vi "Query_SubVIs-某型振动实验台测试系统.vi"(8 "Error":errorcluster) -> (0 "Error":errorcluster)   [LabVIEW 2011]
doc: "Use this template to build a VI to use as a subVI."
uses:
  Ctrls/ana data.ctl
panel:
  out "units":string[](array[string])
  out "粉尘特性":T1
  out "测试条件out":T2
  in  "Tempre Chart 2":waveform(dbl)
  in  "Tempre Chart":waveform(dbl)
  in  "Exit":bool caption="返回"
  in  "Report":bool caption="生成报表"
  in  "Open":bool caption="读取"
  in  "Temp":T3={"Vibr Chn Name"=[], "Analysis Chn Number"=0, "Index Vibration Waveform"={"t0"=timestamp(0 s since 1904-01-01), "dt"=1.0, "Y"=[]}, "Report Infomation"={"Test Name"="", "Tester"="", "Tempre Chart"=refnum, "Apli-Fre"=refnum, "Phase-Fre"=refnum, "Raw Data"=refnum}, "Vibr Apli - Fre"=[], "Vibr Phase - Fre"=[], "Error"={"status"=FALSE, "code"=0, "source"=""}, "Read Chan Name"="", "Test Info"={"Test Name"="", "Tester"=""}, "test data"=[{"t0"=timestamp(0 s since 1904-01-01), "dt"=1.0, "Y"=[]}, {"t0"=timestamp(0 s since 1904-01-01), "dt"=1.0, "Y"=[]}, {"t0"=timestamp(0 s since 1904-01-01), "dt"=1.0, "Y"=[]}, {"t0"=timestamp(0 s since 1904-01-01), "dt"=0.001, "Y"=[]}], "测试头文件"={"ch"=[{"pmax"="", "dp/dt"=""}, {"pmax"="", "dp/dt"=""}, {"pmax"="", "dp/dt"=""}, {"pmax"="", "dp/dt"=""}, {"pmax"="无", "dp/dt"="无"}], "测试环境"=""}, "CAl VAlUE"={"max_t"=[], "max_V"=[], "start_t"=[], "start_V"=[], "distance"=[], "unit"="m"}}
  out "Tester":string caption="实验人"
  out "Test Name":string caption="实验名称"
  in  "Tab Control":enum32{"信号原始数据", "幅频波形", "相频波形"}(tab)
  out "start point":string
  out "high point":string
  in  "unit":enum16{"m", "Km"}(ring) caption="单位："
  in  "print":bool
  out "max_t1":dbl caption="1点至2点"
  out "start_t1":dbl caption="1点至2点"
  out "max_V2":dbl caption="1点至3点"
  out "max_V1":dbl caption="1点至2点"
  in  "T_AN":bool
  out "Raw Data Chart":waveform(dbl)[](graph)
  in  "Tree":string(tree)="PXI-4472/ai0"
  in  "平均时间(S)":dbl=0.002
  in  "Radio Buttons":enum32{"原始数据", "处理数据"}(radio)
  in  "1点至2点距离":dbl=11.0
  in  "1点至3点距离":dbl=12.0
  out "max_t2":dbl caption="1点至3点"
  out "start_t2":dbl caption="1点至3点"
  out "start_V1":dbl caption="1点至2点"
  out "start_V2":dbl caption="1点至3点"
  out "high point 2":string
  out "start point 2":string
  out "Apli-Fre":cluster{dbl, dbl}[](graph)
  out "Phase-Frequency":cluster{dbl, dbl}[](graph)
  # "数据查询与分析"
  # "最高点\n  延迟时间："
  # "s"
  # "s"
  # "最高点\n   传播速度："
  # "开始点\n    延迟时间："
  # "s"
  # "s"
  # "开始点\n   传播速度："
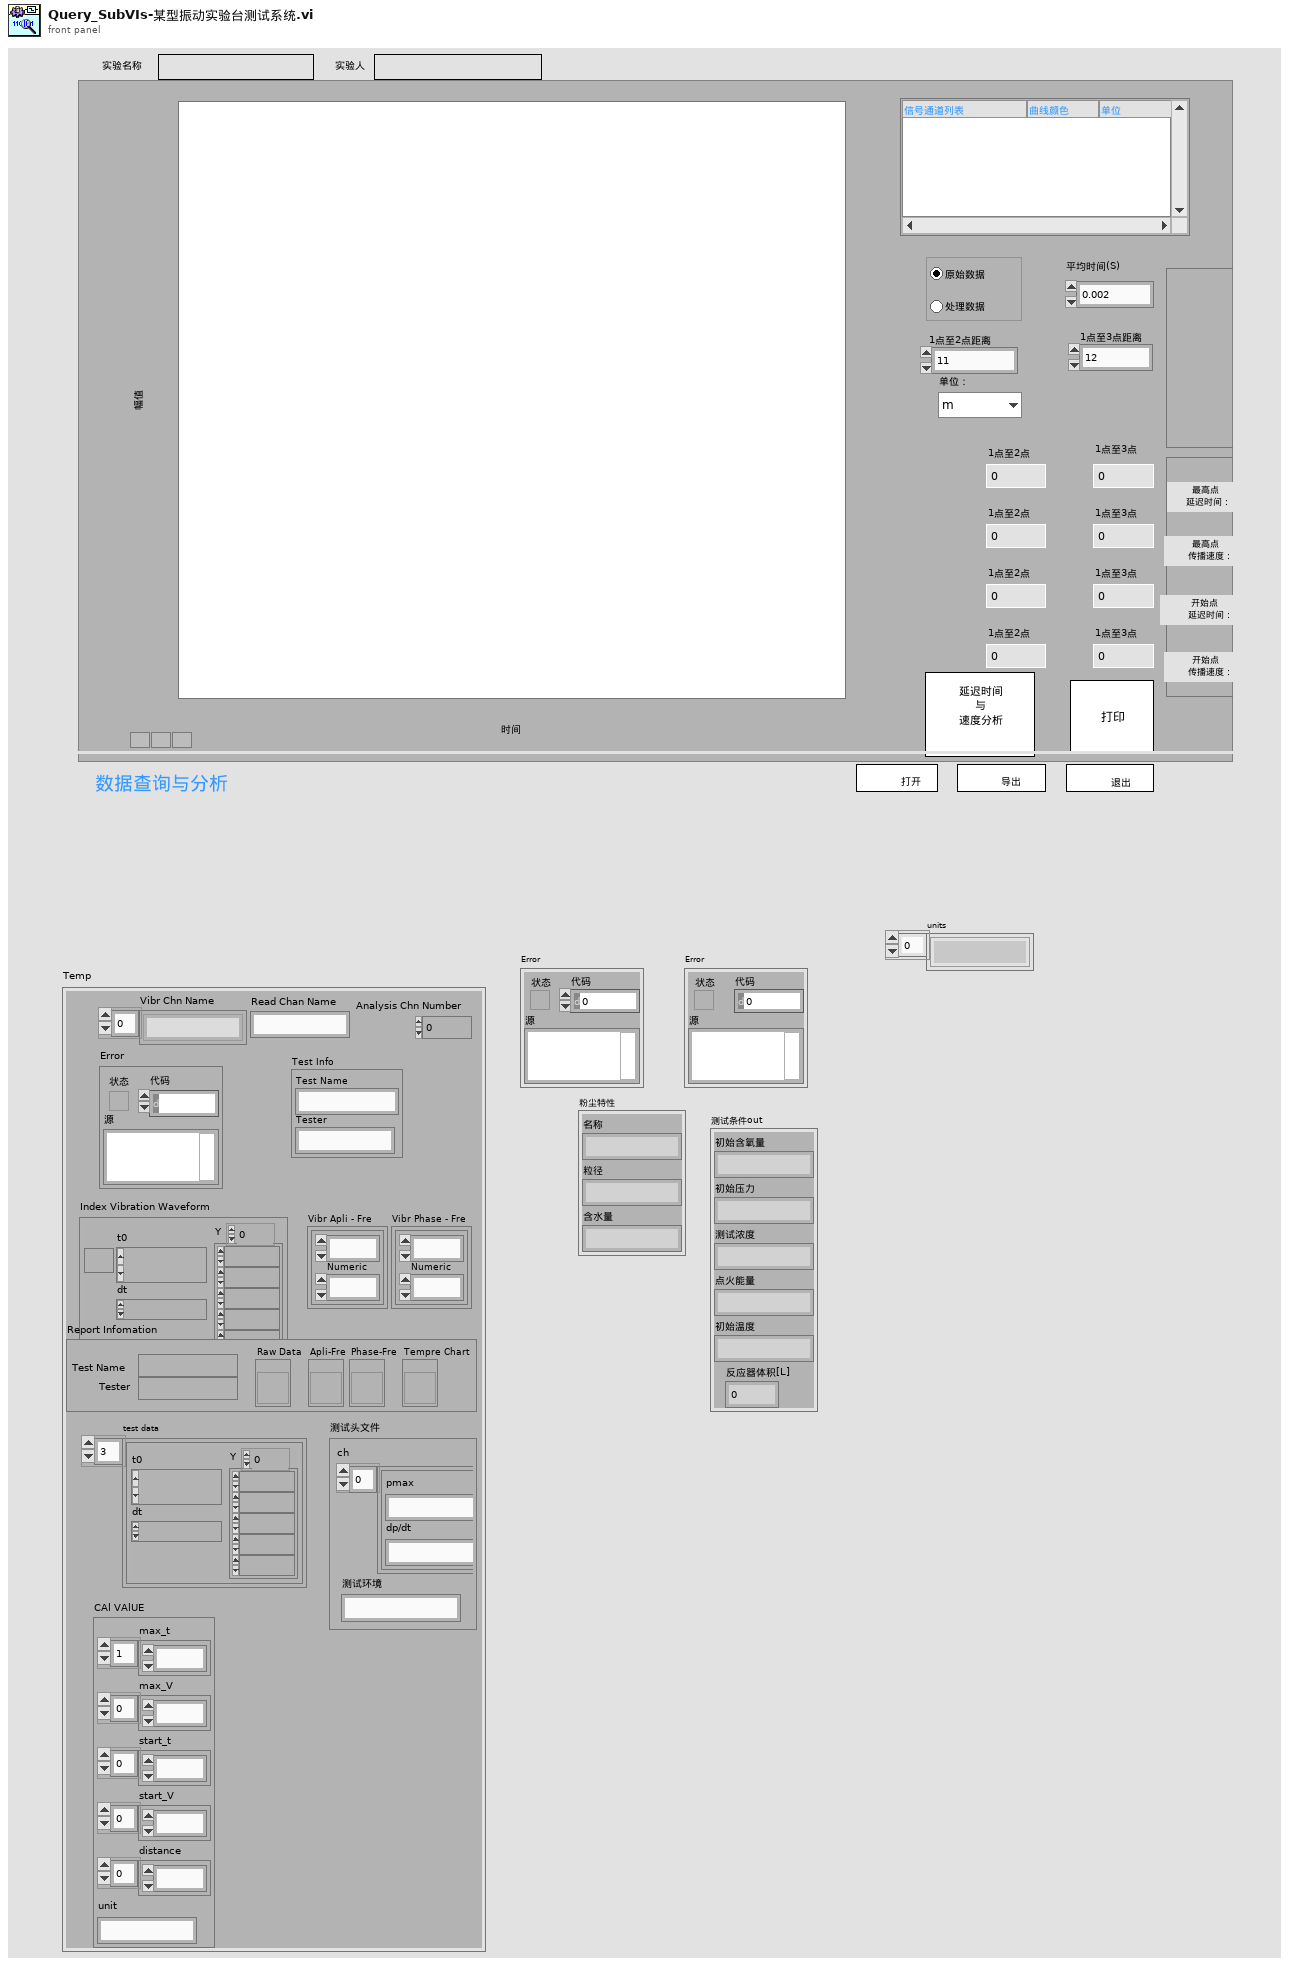
[diagram p1: front panel]
types:
  T1 = typedef "粉尘特性.ctl" = cluster{"名称":string, "粒径":string, "含水量":string}
  T2 = typedef "测试条件.ctl" = cluster{"初始含氧量":string, "初始压力":string, "测试浓度":string, "点火能量":string, "初始温度":string, "反应器体积[L]":dbl}
  T3 = typedef "ana data.ctl" = cluster{"Vibr Chn Name":string[], "Analysis Chn Number":i32, "Index Vibration Waveform":waveform(dbl), "Report Infomation":cluster{"Test Name":string, "Tester":string, "Tempre Chart":refnum<vi>, "Apli-Fre":refnum<vi>, "Phase-Fre":refnum<vi>, "Raw Data":refnum<vi>}, "Vibr Apli - Fre":cluster{dbl, "Numeric":dbl}[], "Vibr Phase - Fre":cluster{dbl, "Numeric":dbl}[], "Error":errorcluster, "Read Chan Name":string, "Test Info":cluster{"Test Name":string, "Tester":string}, "test data":waveform(dbl)[], "测试头文件":cluster{"ch":cluster{"pmax":string, "dp/dt":string}[], "测试环境":string}, "CAl VAlUE":cluster{"max_t":dbl[], "max_V":dbl[], "start_t":dbl[], "start_V":dbl[], "distance":dbl[], "unit":string}}
  T4 = typedef "Enum Query_Ctrls-某型振动实验台测试系统.ctl" = enum16{"Initialize", "No Action", "Open TDMS File", "Read Raw Data", "Analyze Data", "Display Data", "Generate Report", "computer timer", "Error Handle", "Exit"}
  T5 = typedef "Enum File IO - FGV(V)_Ctrls-某型振动实验台测试系统.ctl" = enum16{"New", "Open", "Write Info", "Write Data", "Read Info", "Read Chan Names", "Read Data", "Close", "None"}
  T6 = typedef "imagedata.ctl" = cluster{"image type":i32, "image depth":i32, "image":u8[], "mask":u8[], "colors":u32[], "Rectangle":cluster{"left":i16, "top":i16, "right":i16, "bottom":i16}}
  T7 = cluster{"max_t":dbl[], "max_V":dbl[], "start_t":dbl[], "start_V":dbl[]}
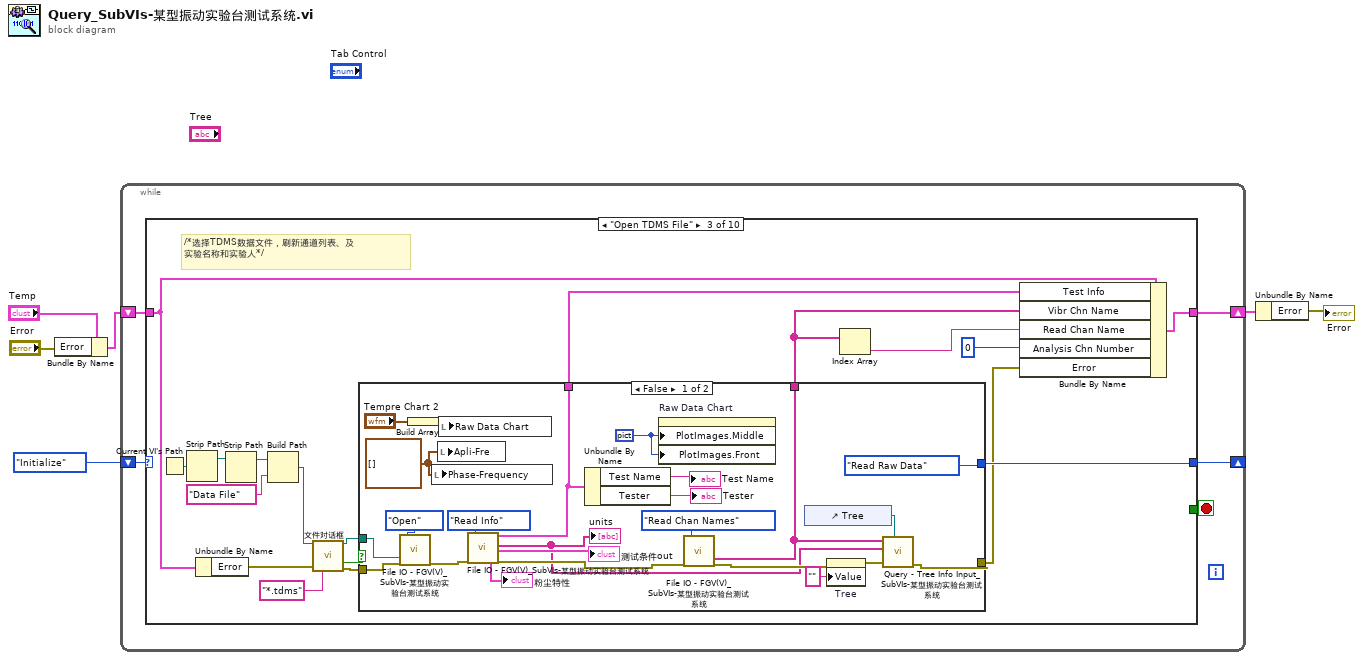
[diagram p0: block diagram]
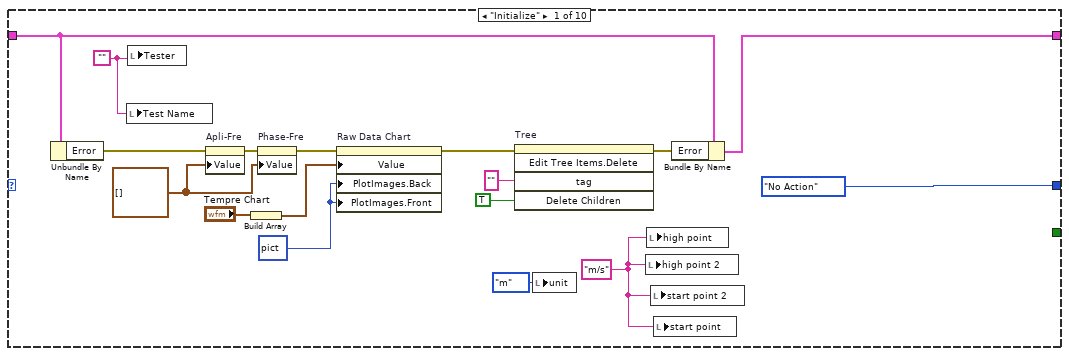
[diagram p2: hidden frame]
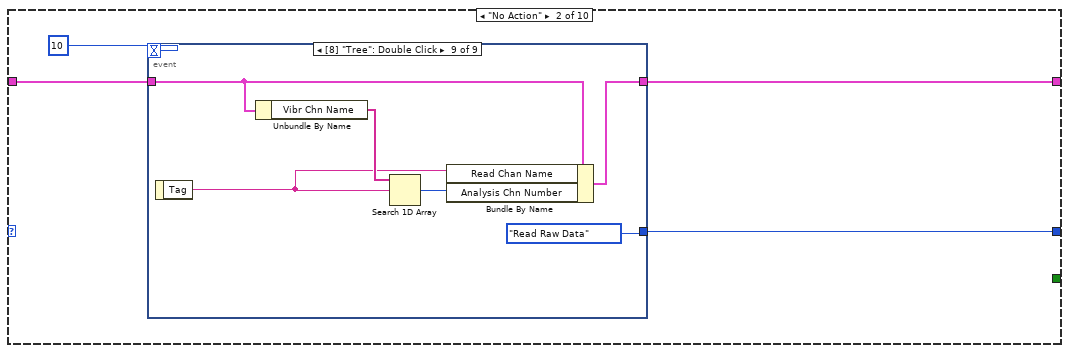
[diagram p3: hidden frame]
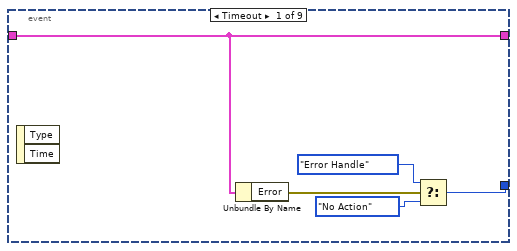
[diagram p4: hidden frame]
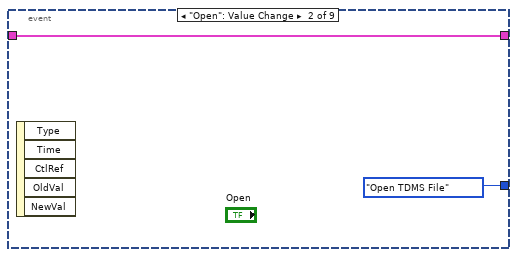
[diagram p5: hidden frame]
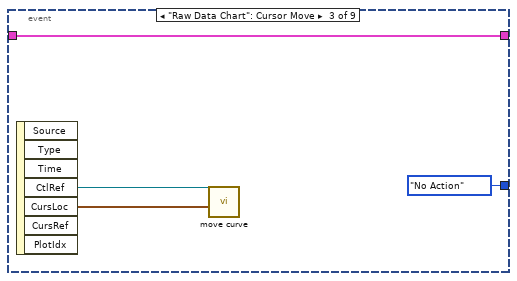
[diagram p6: hidden frame]
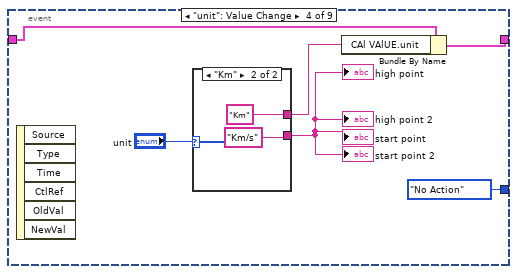
[diagram p7: hidden frame]
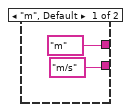
[diagram p8: hidden frame]
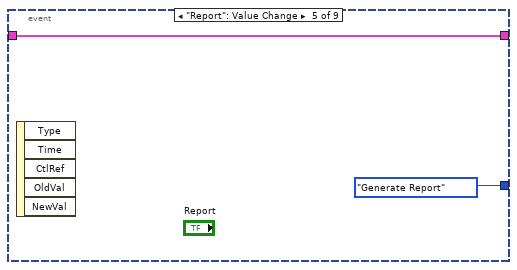
[diagram p9: hidden frame]
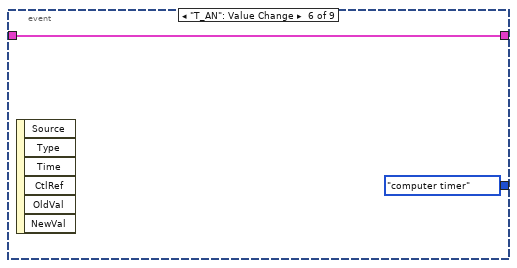
[diagram p10: hidden frame]
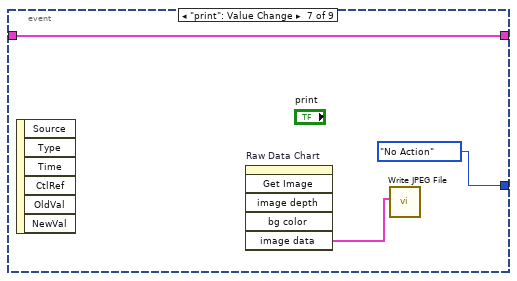
[diagram p11: hidden frame]
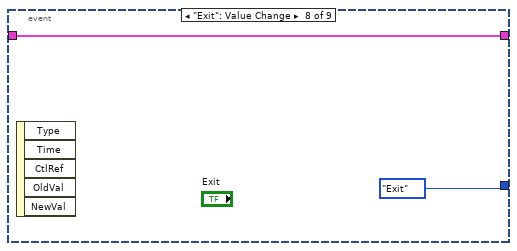
[diagram p12: hidden frame]
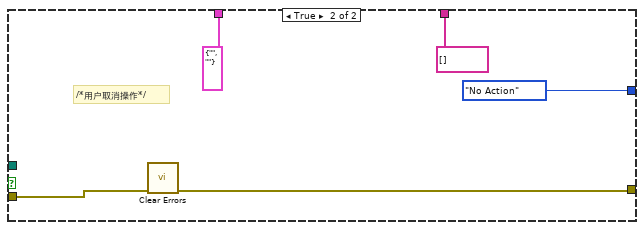
[diagram p13: hidden frame]
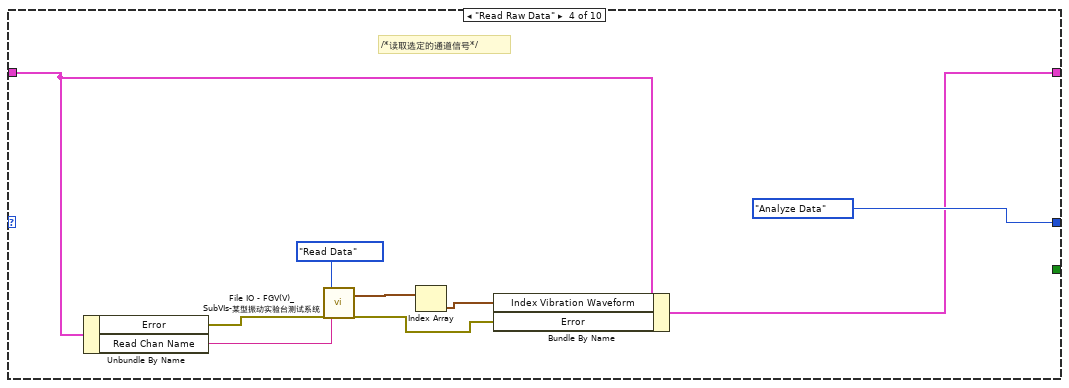
[diagram p14: hidden frame]
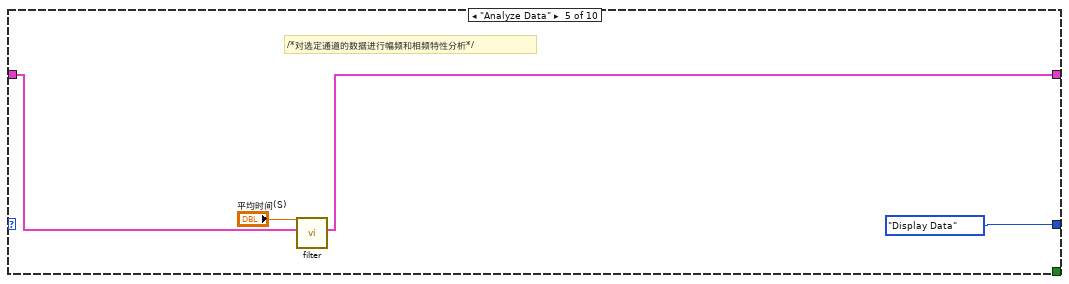
[diagram p15: hidden frame]
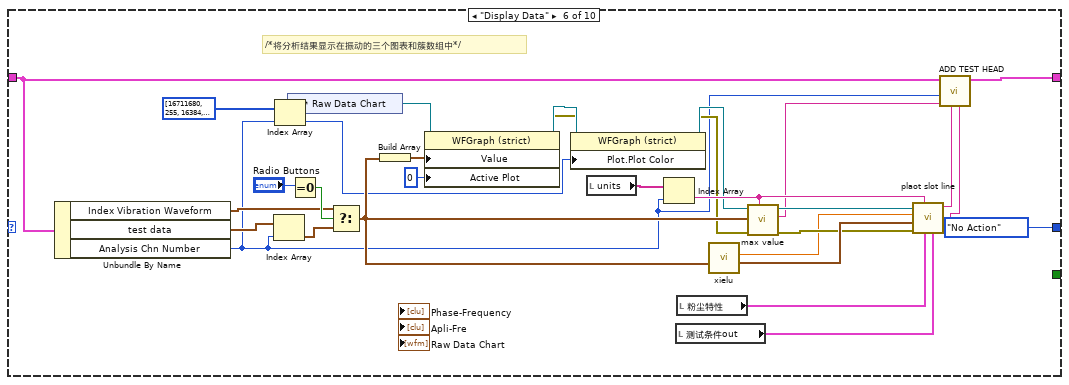
[diagram p16: hidden frame]
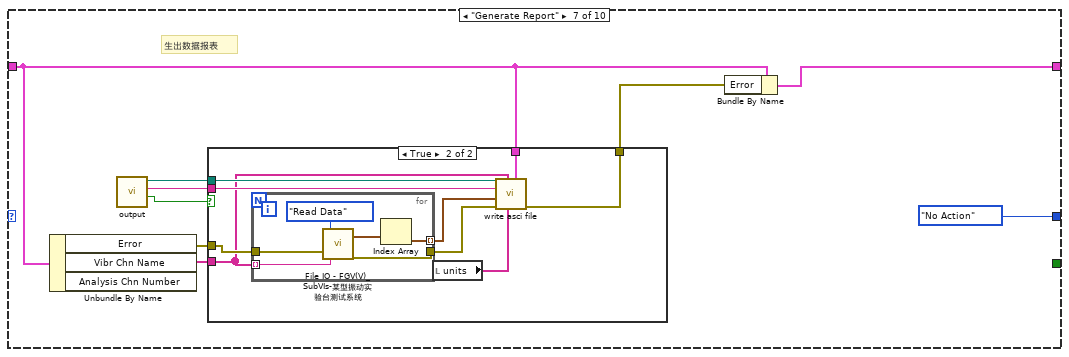
[diagram p17: hidden frame]
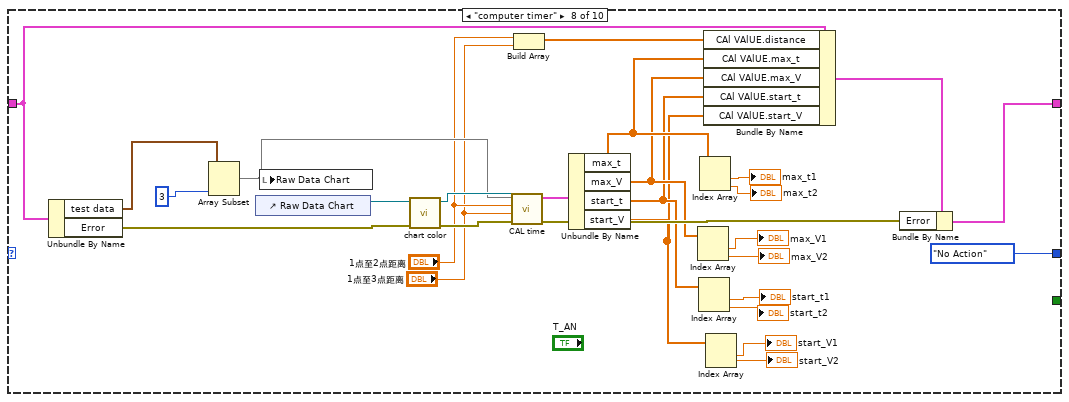
[diagram p19: hidden frame]
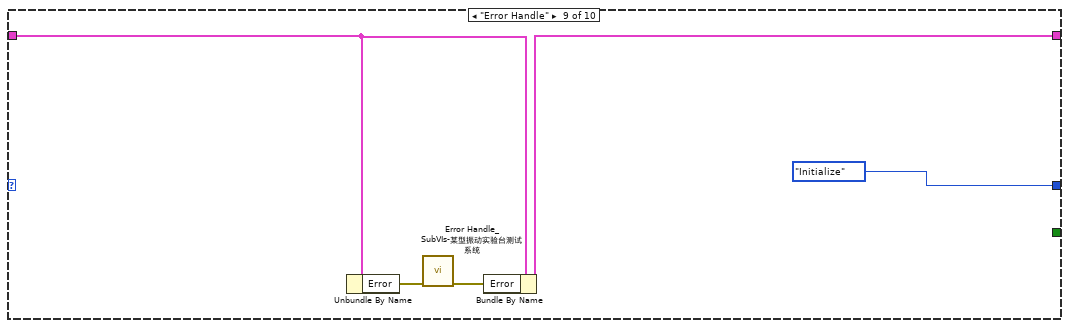
[diagram p20: hidden frame]
diagram:
  n1 = Bundle By Name(cluster="Temp", "Error"="Error") -> (w3:T3)
  n2 = while {
    shift-right: [w10] -> _
    shift-left: Enum_Query_Ctrls-某型振动实验台测试系统."Initialize" ("Enum") -> [w11]
    shift-right: [w7] -> w2
    shift-left: w3 -> [w8]
    stop <- w9 stop-if-true
    n3 = case shown="\"Open TDMS File\"" w11 {
      tunnel: [Enum_Query_Ctrls-某型振动实验台测试系统."No Action" ("Enum") w31 w77 Enum_Query_Ctrls-某型振动实验台测试系统."Analyze Data" ("Enum") Enum_Query_Ctrls-某型振动实验台测试系统."Display Data" ("Enum") Enum_Query_Ctrls-某型振动实验台测试系统."No Action" ("Enum") Enum_Query_Ctrls-某型振动实验台测试系统."No Action" ("Enum") Enum_Query_Ctrls-某型振动实验台测试系统."No Action" ("Enum") Enum_Query_Ctrls-某型振动实验台测试系统."Initialize" ("Enum") Enum_Query_Ctrls-某型振动实验台测试系统."Exit" ("Enum")] -> w10
      tunnel: [_ _ _ _ _ _ _ _ _ TRUE] -> w9
      tunnel: w8 -> [w22 w30 w72 w121 w127 w134 w159 w191 w212 w216]
      tunnel: [w20 w29 w76 w123 w126 w133 w166 w209 w211 w216] -> w7
      frame "Initialize" {
        w14 = picture data[5B] ("曲线图像:前景")
        w12 = "m/s" ("Tag")
        w24 = cluster{dbl, dbl}[] [] ("Aplitude-Frequency")
        w25 = ""
        n4 = Unbundle By Name(w22) -> ("Error"=w23:errorcluster)
        n5 = local write "Test Name"(w25) -> ()
        n6 = local write "Tester"(w25) -> ()
        n7 = property on="Apli-Fre" class="XYGraph (strict)"(error in=w23, "Value"=w24) -> (error out=w27:errorcluster)  [unwired: 1 in, 1 out]
        n8 = Build Array("Tempre Chart") -> (w15:waveform(dbl)[])
        n9 = property on="Phase-Fre" class="XYGraph (strict)"(error in=w27, "Value"=w24) -> (error out=w26:errorcluster)  [unwired: 1 in, 1 out]
        n10 = property on="Raw Data Chart" class="WFGraph (strict)"(error in=w26, "Value"=w15, "PlotImages.Back"=w14, "PlotImages.Front"=w14) -> (error out=w19:errorcluster)  [unwired: 1 in, 1 out]
        n11 = invoke on="Tree" class="Tree (严格)" method="Edit Tree Items.Delete"(error in=w19, "tag"="" ("Tag"), "Delete Children"=TRUE ("Delete Children?")) -> (error out=w21:errorcluster)  [unwired: 2 in, 4 out]
        n12 = local write "unit"(enum16{"m", "Km"}."m" ("unit")) -> ()
        n13 = local write "high point 2"(w12) -> ()
        n14 = local write "high point"(w12) -> ()
        n15 = local write "start point 2"(w12) -> ()
        n16 = local write "start point"(w12) -> ()
        n17 = Bundle By Name(cluster=w22, "Error"=w21) -> (w20:T3)
      }
      frame "No Action" {
        n18 = event shown="[8] \"Tree\": Double Click" {
          selector: _ -> [_ _ _ _ _ _ _ _ _]
          dyn-events: _ -> [_ _ _ _ _ _ _ _ _]
          timeout: 10 -> [_ _ _ _ _ _ _ _ _]
          tunnel: [w35 Enum_Query_Ctrls-某型振动实验台测试系统."Open TDMS File" ("Enum") Enum_Query_Ctrls-某型振动实验台测试系统."No Action" ("Enum") Enum_Query_Ctrls-某型振动实验台测试系统."No Action" ("Enum") Enum_Query_Ctrls-某型振动实验台测试系统."Generate Report" ("Enum") Enum_Query_Ctrls-某型振动实验台测试系统."computer timer" ("Enum") Enum_Query_Ctrls-某型振动实验台测试系统."No Action" ("Enum") Enum_Query_Ctrls-某型振动实验台测试系统."Exit" ("Enum") Enum_Query_Ctrls-某型振动实验台测试系统."Read Raw Data" ("Enum")] -> w31
          tunnel: w30 -> [w34 w38 w43 w46 w54 w57 w60 w61 w65]
          tunnel: [w34 w38 w43 w45 w54 w57 w60 w61 w64] -> w29
          event Timeout {
            n19 = event-data() -> ()  [unwired: 3 out]
            n20 = Unbundle By Name(w34) -> ("Error"=w33:errorcluster)
            n21 = Select(t=Enum_Query_Ctrls-某型振动实验台测试系统."Error Handle" ("Enum"), s=w33, f=Enum_Query_Ctrls-某型振动实验台测试系统."No Action" ("Enum")) -> (s? t:f=w35:T4)
          }
          event "Open": Value Change {
            n22 = event-data() -> ()  [unwired: 6 out]
          }
          event "Raw Data Chart": Cursor Move {
            n23 = event-data() -> ("CtlRef"=w41:refnum<vi>, "CursLoc"=w40:cluster{"X":dbl, "Y":dbl})  [unwired: 6 out]
            n24 = call "move curve.vi"("XY"=w40, "引用"=w41) -> ()  [unwired: 1 in, 9 out]
          }
          event "unit": Value Change {
            n25 = event-data() -> ()  [unwired: 7 out]
            n26 = case shown="\"Km\"" "unit" {
              tunnel: ["m/s" "Km/s"] -> w47
              tunnel: ["m" "Km"] -> w44
              frame "m", Default {
              }
              frame "Km" {
              }
            }
            "high point" <- w47
            "start point" <- w47
            "high point 2" <- w47
            "start point 2" <- w47
            n27 = Bundle By Name(cluster=w46, "CAl VAlUE.unit"=w44) -> (w45:T3)
          }
          event "Report": Value Change {
            n28 = event-data() -> ()  [unwired: 6 out]
          }
          event "T_AN": Value Change {
            n29 = event-data() -> ()  [unwired: 7 out]
          }
          event "print": Value Change {
            n30 = event-data() -> ()  [unwired: 7 out]
            n31 = invoke on="Raw Data Chart" class="WFGraph (严格)" method="Get Image"() -> ("image data"=w59:T6)  [unwired: 6 in, 5 out]
            n32 = call <vilib>:"Write JPEG File.vi"("image data"=w59) -> ()  [unwired: 2 in, 9 out]
          }
          event "Exit": Value Change {
            n33 = event-data() -> ()  [unwired: 6 out]
          }
          event "Tree": Double Click {
            n34 = event-data() -> ("Tag"=w63:string)  [unwired: 1 out]
            n35 = Unbundle By Name(w65) -> ("Vibr Chn Name"=w67:string[])
            n36 = Search 1D Array(1D array=w67, element=w63) -> (index of element=w66:i32)  [unwired: 1 out]
            n37 = Bundle By Name(cluster=w65, "Read Chan Name"=w63, "Analysis Chn Number"=w66) -> (w64:T3)
          }
        }
      }
      frame "Open TDMS File" {
        # "/*选择TDMS数据文件，刷新通道列表、及\n实验名称和实验人*/"
        n38 = Current VI's Path() -> (path=w82:path)
        n39 = Strip Path(path=w82) -> (stripped path=w83:path)  [unwired: 1 out]
        n40 = Unbundle By Name(w72) -> ("Error"=w74:errorcluster)
        n41 = Strip Path(path=w83) -> (stripped path=w81:path)  [unwired: 1 out]
        n42 = Build Path(base path=w81, name or relative path="Data File") -> (appended path=w78:path)
        n43 = call "文件对话框"("start path"=w78, "error in"=w74, "pattern (all files)"="*.tdms") -> ("selected path"=w86:path, "cancelled"=w84:bool, "error out"=w85:errorcluster)  [unwired: 4 in, 6 out]
        n44 = case shown="False" w84 {
          tunnel: w86 -> [w101 _]
          tunnel: [w87 w115] -> w73
          tunnel: w85 -> [w100 w114]
          tunnel: [w105 string[] [] ("Vibration Channel Name Output")] -> w70
          tunnel: [Enum_Query_Ctrls-某型振动实验台测试系统."Read Raw Data" ("Enum") Enum_Query_Ctrls-某型振动实验台测试系统."No Action" ("Enum")] -> w77
          tunnel: [w96 cluster{"Test Name":string, "Tester":string} {"Test Name"="", "Tester"=""} ("Name")] -> w75
          frame False {
            w91 = picture data[5B] ("曲线图像:背景")
            w102 = cluster{dbl, dbl}[] [] ("Aplitude-Frequency")
            n45 = call "File IO - FGV(V)_SubVIs-某型振动实验台测试系统.vi"("文件路径"=w101, "error in"=w100, "Operation"=Enum_File_IO_-_FGV(V)_Ctrls-某型振动实验台测试系统."Open") -> ("error out"=w98:errorcluster)  [unwired: 7 in, 9 out]
            n46 = Build Array("Tempre Chart 2") -> (w94:waveform(dbl)[])
            n47 = local write "Phase-Frequency"(w102) -> ()
            n48 = local write "Apli-Fre"(w102) -> ()
            n49 = local write "Raw Data Chart"(w94) -> ()
            n50 = call "File IO - FGV(V)_SubVIs-某型振动实验台测试系统.vi"("error in"=w98, "Operation"=Enum_File_IO_-_FGV(V)_Ctrls-某型振动实验台测试系统."Read Info") -> ("粉尘特性 out"=→"粉尘特性":T1, "Test Info"=w96:cluster{"Test Name":string, "Tester":string}, "units"=w89:string[], "测试条件out"=→"测试条件out":T2, "error out"=w99:errorcluster)  [unwired: 8 in, 5 out]
            "units" <- w89
            n51 = Unbundle By Name(w96) -> ("Test Name"=→"Test Name":string, "Tester"=→"Tester":string)
            n52 = property on="Raw Data Chart" class="WFGraph (strict)"("PlotImages.Middle"=w91, "PlotImages.Front"=w91) -> ()  [unwired: 2 in, 2 out]
            n53 = call "File IO - FGV(V)_SubVIs-某型振动实验台测试系统.vi"("error in"=w99, "Operation"=Enum_File_IO_-_FGV(V)_Ctrls-某型振动实验台测试系统."Read Chan Names") -> ("Vibration Chan Names Out"=w105:string[], "error out"=w106:errorcluster)  [unwired: 8 in, 8 out]
            n54 = control-ref of="Tree"() -> (w88:refnum<vi>)
            n55 = property on="Tree" class="Tree (strict)"(error in=w106, "Value"="" ("Tree")) -> (error out=w90:errorcluster)  [unwired: 1 in, 1 out]
            n56 = call "Query - Tree Info Input_SubVIs-某型振动实验台测试系统.vi"("Tree引用句柄"=w88, "错误输入（无错误）"=w90, "units"=w89, "Vibration Channel Name Output"=w105) -> ("错误输出"=w87:errorcluster)  [unwired: 7 out]
          }
          frame True {
            # "/*用户取消操作*/"
            n57 = call <vilib>:"Clear Errors.vi"("error in (no error)"=w114) -> ("error out"=w115:errorcluster)  [unwired: 6 out]
          }
        }
        n58 = Index Array(array=w70) -> (element=w71:string)  [unwired: 1 in]
        n59 = Bundle By Name(cluster=w72, "Test Info"=w75, "Vibr Chn Name"=w70, "Read Chan Name"=w71, "Analysis Chn Number"=0, "Error"=w73) -> (w76:T3)
      }
      frame "Read Raw Data" {
        # "/*读取选定的通道信号*/"
        n60 = Unbundle By Name(w121) -> ("Error"=w120:errorcluster, "Read Chan Name"=w116:string)
        n61 = call "File IO - FGV(V)_SubVIs-某型振动实验台测试系统.vi"("error in"=w120, "Operation"=Enum_File_IO_-_FGV(V)_Ctrls-某型振动实验台测试系统."Read Data", "Chan"=w116) -> ("Vibration Waveform"=w118:waveform(dbl)[], "error out"=w119:errorcluster)  [unwired: 7 in, 8 out]
        n62 = Index Array(array=w118) -> (element=w122:waveform(dbl))  [unwired: 1 in]
        n63 = Bundle By Name(cluster=w121, "Index Vibration Waveform"=w122, "Error"=w119) -> (w123:T3)
      }
      frame "Analyze Data" {
        # "/*对选定通道的数据进行幅频和相频特性分析*/"
        n64 = call "filter.vi"("Temp"=w127, "averaging time"="平均时间(S)") -> ("Temp out"=w126:T3)  [unwired: 2 in, 7 out]
      }
      frame "Display Data" {
        # "/*将分析结果显示在振动的三个图表和簇数组中*/"
        n65 = Unbundle By Name(w134) -> ("Index Vibration Waveform"=w156:waveform(dbl), "test data"=w155:waveform(dbl)[], "Analysis Chn Number"=w132:i32)
        n66 = Index Array(array=w155, index=w132) -> (element=w154:waveform(dbl))
        n67 = Index Array(array=u32[] [16711680, 255, 16384, 4194432, 16750848], index=w132) -> (element=w139:u32)
        n68 = control-ref of="Raw Data Chart"() -> (w141:refnum<vi>)
        n69 = Equal To 0?(x="Radio Buttons") -> (x = 0?=w157:bool)
        n70 = Select(t=w156, s=w157, f=w154) -> (s? t:f=w153:waveform(dbl))
        n71 = Build Array(w153) -> (w143:waveform(dbl)[])
        n72 = property class="WFGraph (strict)"(reference=w141, "Value"=w143, "Active Plot"=u32 0 ("活动曲线")) -> (reference out=w140:refnum<vi>, error out=w136:errorcluster)  [unwired: 1 in]
        n73 = property class="WFGraph (strict)"(reference=w140, error in=w136, "Plot.Plot Color"=w139) -> (reference out=w138:refnum<vi>, error out=w137:errorcluster)
        n74 = local read "units"() -> (w149:string[])
        n75 = Index Array(array=w149, index=w132) -> (element=w148:string)
        n76 = local read "测试条件out"() -> (w146:T2)
        n77 = local read "粉尘特性"() -> (w147:T1)
        n78 = call "xielu.vi"("waveform in"=w153) -> ("plot site"=w152:cluster{"X":dbl, "Y":dbl}[], "slop max value"=w150:dbl)  [unwired: 5 out]
        n79 = call "max value.vi"("unit"=w148, "error in (no error)"=w137, "waveform in"=w153, "Raw refum"=w138) -> ("error out"=w151:errorcluster, "Pmax"=w131:string, "引用输出"=w142:refnum<vi>)  [unwired: 5 out]
        n80 = call "plaot slot line.vi"("测试条件out"=w146, "粉尘特性"=w147, "unit"=w148, "error in (no error)"=w151, "max slop value"=w152, "max slop"=w150, "plot graph"=w142) -> ("测试条件"=w129:string, "dp/dt"=w130:string)  [unwired: 3 out]
        n81 = call "ADD TEST HEAD.vi"("测试头文件.测试环境"=w129, "dp/dt"=w130, "pmax"=w131, "ch no"=w132, "Temp in"=w134) -> ("Temp out"=w133:T3)  [unwired: 6 out]
      }
      frame "Generate Report" {
        # "生出数据报表"
        n82 = Unbundle By Name(w159) -> ("Error"=w165:errorcluster, "Vibr Chn Name"=w162:string[])  [unwired: 1 out]
        n83 = call "output.vi"() -> ("ok?"=w160:bool, "txt?excel"=w163:string, "path"=w164:path)  [unwired: 9 out]
        n84 = case shown="True" w160 {
          tunnel: w165 -> [_ w176]
          tunnel: w164 -> [_ w175]
          tunnel: w163 -> [_ w174]
          tunnel: w162 -> [_ w173]
          tunnel: [_ w170] -> w161
          tunnel: w159 -> [_ w168]
          frame False {
          }
          frame True {
            n85 = for {
              tunnel: w173 -> [w180] mode=indexing
              tunnel: [w178] -> w172 mode=indexing
              tunnel: w176 -> [w182]
              tunnel: [w177] -> w171
              n86 = call "File IO - FGV(V)_SubVIs-某型振动实验台测试系统.vi"("error in"=w182, "Operation"=Enum_File_IO_-_FGV(V)_Ctrls-某型振动实验台测试系统."Read Data", "Chan"=w180) -> ("Vibration Waveform"=w179:waveform(dbl)[], "error out"=w177:errorcluster)  [unwired: 7 in, 8 out]
              n87 = Index Array(array=w179) -> (element=w178:waveform(dbl))  [unwired: 1 in]
            }
            n88 = local read "units"() -> (w169:string[])
            n89 = call "write asci file.vi"("Temp in"=w168, "unit"=w169, "chanel name"=w173, "error in (no error)"=w171, "data"=w172, "格式"=w174, "file (use dialog)"=w175) -> ("error out"=w170:errorcluster)  [unwired: 4 out]
          }
        }
        n90 = Bundle By Name(cluster=w159, "Error"=w161) -> (w166:T3)
      }
      frame "computer timer" {
        n91 = Unbundle By Name(w191) -> ("test data"=w207:waveform(dbl)[], "Error"=w194:errorcluster)
        n92 = Array Subset(array=w207, length=3) -> (w192:waveform(dbl)[])  [unwired: 1 in]
        n93 = control-ref of="Raw Data Chart"() -> (w196:refnum<vi>)
        n94 = local write "Raw Data Chart"(w192) -> ()
        n95 = call "chart color.vi"("错误输入（无错误）"=w194, "Chart ref in"=w196) -> ("错误输出"=w193:errorcluster, "Chart ref out"=w195:refnum<vi>)  [unwired: 8 out]
        n96 = call "CAL time.vi"("reference"=w195, "error in (no error)"=w193, "S2"="1点至3点距离", "S1"="1点至2点距离", "appended array"=w192) -> ("error out"=w208:errorcluster, "CAl VAlUE"=w205:T7)  [unwired: 5 out]
        n97 = Build Array("1点至2点距离", "1点至3点距离") -> (w187:dbl[])
        n98 = Unbundle By Name(w205) -> ("max_t"=w186:dbl[], "max_V"=w185:dbl[], "start_t"=w184:dbl[], "start_V"=w183:dbl[])
        n99 = Index Array(array=w185) -> (element #1=→"max_V1":dbl, element #2=→"max_V2":dbl)  [unwired: 2 in]
        n100 = Index Array(array=w184) -> (element #1=→"start_t1":dbl, element #2=→"start_t2":dbl)  [unwired: 2 in]
        n101 = Index Array(array=w186) -> (element #1=→"max_t1":dbl, element #2=→"max_t2":dbl)  [unwired: 2 in]
        n102 = Bundle By Name(cluster=w191, "CAl VAlUE.distance"=w187, "CAl VAlUE.max_t"=w186, "CAl VAlUE.max_V"=w185, "CAl VAlUE.start_t"=w184, "CAl VAlUE.start_V"=w183) -> (w190:T3)
        n103 = Index Array(array=w183) -> (element #1=→"start_V1":dbl, element #2=→"start_V2":dbl)  [unwired: 2 in]
        n104 = Bundle By Name(cluster=w190, "Error"=w208) -> (w209:T3)
      }
      frame "Error Handle" {
        n105 = Unbundle By Name(w212) -> ("Error"=w214:errorcluster)
        n106 = call "Error Handle_SubVIs-某型振动实验台测试系统.vi"("error in"=w214) -> ("error out"=w213:errorcluster)  [unwired: 10 out]
        n107 = Bundle By Name(cluster=w212, "Error"=w213) -> (w211:T3)
      }
      frame "Exit" {
      }
    }
  }
  n108 = Unbundle By Name(w2) -> ("Error"=→"Error":errorcluster)
